vi "DMM Resistance Meas Format Function Range.vi"(0 "DMM Handle In":refnum<k15>, 5 "Function Settings In":T1={"Range and Function"=enum."2w-Resistance Auto Range", "Resolution in Digits"=5.5} {"Resolution in Digits" items=["3 1/2"=3.5, "4 1/2"=4.5, "5 1/2"=5.5, "6 1/2"=6.5, "7 1/2"=7.5]}, 11 "error in":errorcluster) -> (4 "DMM Handle Out":refnum<k15>, 6 "Function Settings Out":T4={"Range"=0.0, "Function"=enum."2-wire Resistance", "AC Range"=0.0, "Resolution in Digits"=5.5} {"Resolution in Digits" items=["3 1/2"=3.5, "4 1/2"=4.5, "5 1/2"=5.5, "6 1/2"=6.5, "7 1/2"=7.5]}, 15 "error out":errorcluster)   [LabVIEW 2021, in "DMM_Resistance Measurement.lvlib"]
doc: "Utilizes the function settings input to select the particular function and range used for the measurement and format the output string displayed in the measurement output cluster."
uses:
  DMM_Resistance Measurement.lvlib
  <instrlib>/niDMM/nidmm.llb/niDMM Function.ctl
  <instrlib>/niDMM/nidmm.llb/niDMM Resolution in Digits.ctl
  DMM Resistance Typedefs/Function Settings.ctl
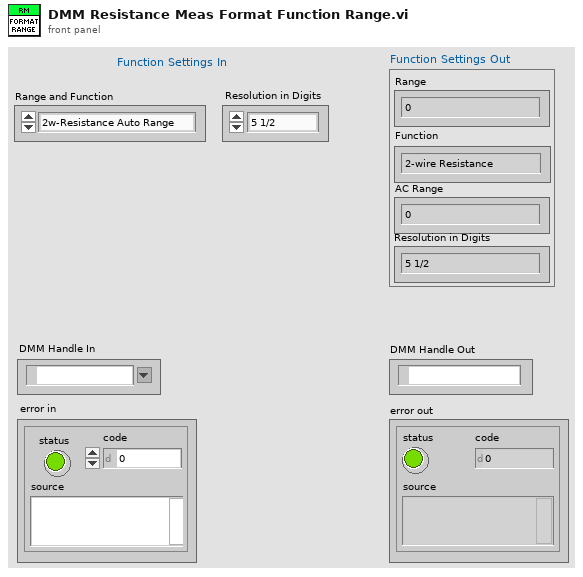
[diagram p1: front panel]
types:
  T1 = typedef "DMM_Resistance Measurement.lvlib/Function Settings.ctl" = cluster{"Range and Function":enum16{"2w-Resistance Auto Range", "2w-Res 100 Ohm", "2w-Res 1 kOhm", "2w-Res 10 kOhm", "2w-Res 100 kOhm", "2w-Res 1 MOhm", "2w-Res 10 MOhm", "2w-Res 100 MOhm", "2w-Res 5 GOhm", "     ", "4w-Resistance Auto Range", "4w-Res 100 Ohm", "4w-Res 1 kOhm", "4w-Res 10 kOhm", "4w-Res 100 kOhm", "4w-Res 1 MOhm", "4w-Res 10 MOhm"}, "Resolution in Digits":T2}
  T2 = typedef "niDMM Resolution in Digits.ctl" = dbl
  T3 = typedef "niDMM Function.ctl" = enum16{"DC Volts", "AC Volts", "DC Current", "AC Current", "2-wire Resistance", "4-wire Resistance", "Diode", "Frequency", "Period", "AC Volts DC Coupled", "Capacitance", "Inductance", "Temperature"}
  T4 = cluster{"Range":dbl, "Function":T3, "AC Range":dbl, "Resolution in Digits":T2}
  T5 = cluster{"Range":dbl, "Function":T3, "Freq_Period AC Range":dbl, "Resolution in Digits":T2}
  T6 = enum16{"2w-Resistance Auto Range", "2w-Res 100 Ohm", "2w-Res 1 kOhm", "2w-Res 10 kOhm", "2w-Res 100 kOhm", "2w-Res 1 MOhm", "2w-Res 10 MOhm", "2w-Res 100 MOhm", "2w-Res 5 GOhm", "     ", "4w-Resistance Auto Range", "4w-Res 100 Ohm", "4w-Res 1 kOhm", "4w-Res 10 kOhm", "4w-Res 100 kOhm", "4w-Res 1 MOhm", "4w-Res 10 MOhm"}
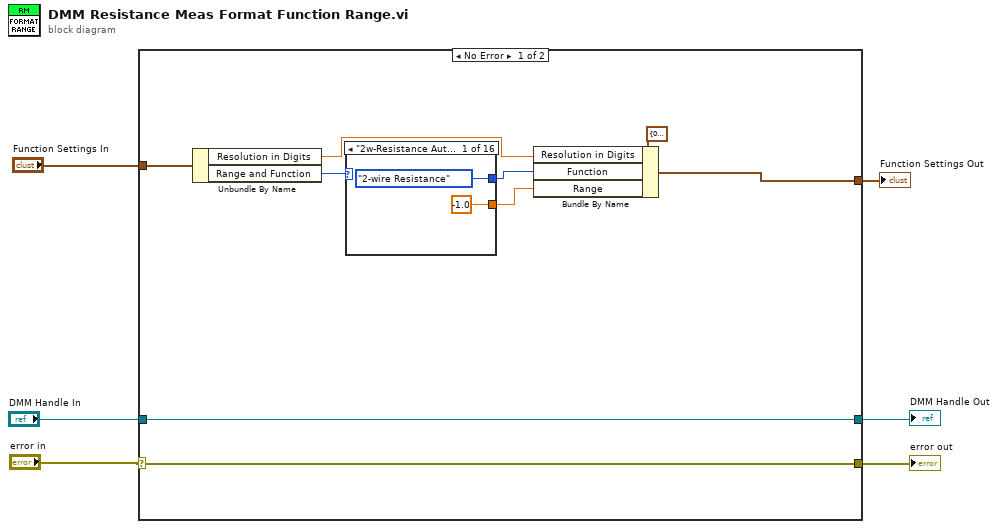
[diagram p0: block diagram]
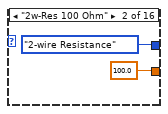
[diagram p2: hidden frame]
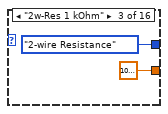
[diagram p3: hidden frame]
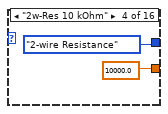
[diagram p4: hidden frame]
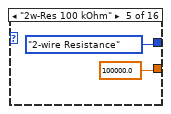
[diagram p5: hidden frame]
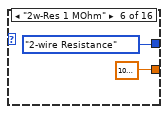
[diagram p6: hidden frame]
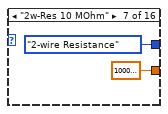
[diagram p7: hidden frame]
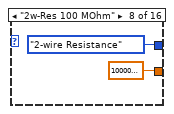
[diagram p8: hidden frame]
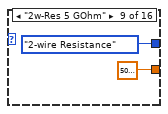
[diagram p9: hidden frame]
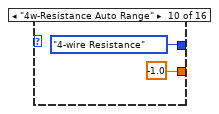
[diagram p10: hidden frame]
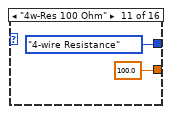
[diagram p11: hidden frame]
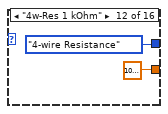
[diagram p12: hidden frame]
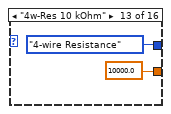
[diagram p13: hidden frame]
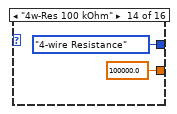
[diagram p14: hidden frame]
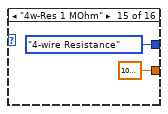
[diagram p15: hidden frame]
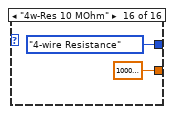
[diagram p16: hidden frame]
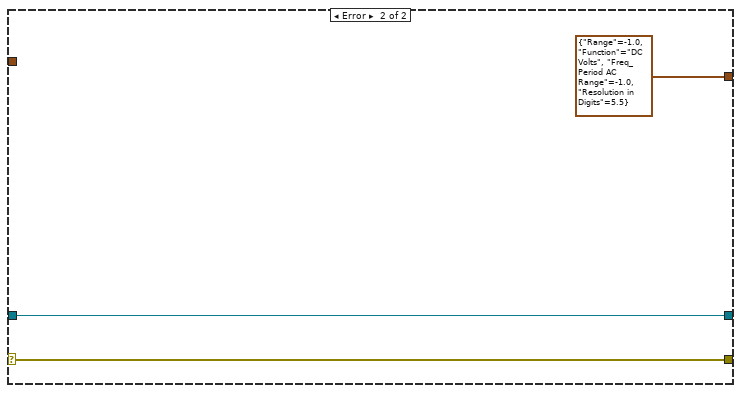
[diagram p17: hidden frame]
diagram:
  n1 = case shown="No Error" "error in" {
    selector: "error in" -> [w8 w49]
    tunnel: "Function Settings In" -> [w15 _]
    tunnel: [w9 T5 {"Range"=-1.0, "Function"=enum."DC Volts", "Freq_Period AC Range"=-1.0, "Resolution in Digits"=5.5} ("Function Settings")] -> w2
    tunnel: [w8 w49] -> w5
    tunnel: [w7 w50] -> w3
    tunnel: "DMM Handle In" -> [w7 w50]
    frame No Error {
      n2 = Unbundle By Name(w15) -> ("Resolution in Digits"=w13:T2, "Range and Function"=w14:T6)
      n3 = case shown="\"2w-Resistance Auto Range\", Default" w14 {
        tunnel: [niDMM_Function."2-wire Resistance" ("Function") niDMM_Function."2-wire Resistance" ("Function") niDMM_Function."2-wire Resistance" ("Function") niDMM_Function."2-wire Resistance" ("Function") niDMM_Function."2-wire Resistance" ("Function") niDMM_Function."2-wire Resistance" ("Function") niDMM_Function."2-wire Resistance" ("Function") niDMM_Function."2-wire Resistance" ("Function") niDMM_Function."2-wire Resistance" ("Function") niDMM_Function."4-wire Resistance" ("Function") niDMM_Function."4-wire Resistance" ("Function") niDMM_Function."4-wire Resistance" ("Function") niDMM_Function."4-wire Resistance" ("Function") niDMM_Function."4-wire Resistance" ("Function") niDMM_Function."4-wire Resistance" ("Function") niDMM_Function."4-wire Resistance" ("Function")] -> w10
        tunnel: [-1.0 ("Range") 100.0 ("Range") 1000.0 ("Range") 10000.0 ("Range") 100000.0 ("Range") 1000000.0 ("Range") 10000000.0 ("Range") 100000000.0 ("Range") 5000000000.0 ("Range") -1.0 ("Range") 100.0 ("Range") 1000.0 ("Range") 10000.0 ("Range") 100000.0 ("Range") 1000000.0 ("Range") 10000000.0 ("Range")] -> w11
        frame "2w-Resistance Auto Range", Default {
        }
        frame "2w-Res 100 Ohm" {
        }
        frame "2w-Res 1 kOhm" {
        }
        frame "2w-Res 10 kOhm" {
        }
        frame "2w-Res 100 kOhm" {
        }
        frame "2w-Res 1 MOhm" {
        }
        frame "2w-Res 10 MOhm" {
        }
        frame "2w-Res 100 MOhm" {
        }
        frame "2w-Res 5 GOhm" {
        }
        frame "4w-Resistance Auto Range" {
        }
        frame "4w-Res 100 Ohm" {
        }
        frame "4w-Res 1 kOhm" {
        }
        frame "4w-Res 10 kOhm" {
        }
        frame "4w-Res 100 kOhm" {
        }
        frame "4w-Res 1 MOhm" {
        }
        frame "4w-Res 10 MOhm" {
        }
      }
      n4 = Bundle By Name(cluster=T5 {"Range"=0.1, "Function"=enum."DC Volts", "Freq_Period AC Range"=0.1, "Resolution in Digits"=5.5} ("Function Settings"), "Resolution in Digits"=w13, "Function"=w10, "Range"=w11) -> (w9:T5)
    }
    frame Error {
    }
  }
  "error out" <- w5
  "DMM Handle Out" <- w3
  "Function Settings Out" <- w2
